vi "Start and Stop Sift Proxy.vi"() -> ()   [LabVIEW 2024]
uses:
  Sift API/Sift Client.lvclass
panel:
  out "Success":bool
  out "Count":i32
  out "Error":errorcluster
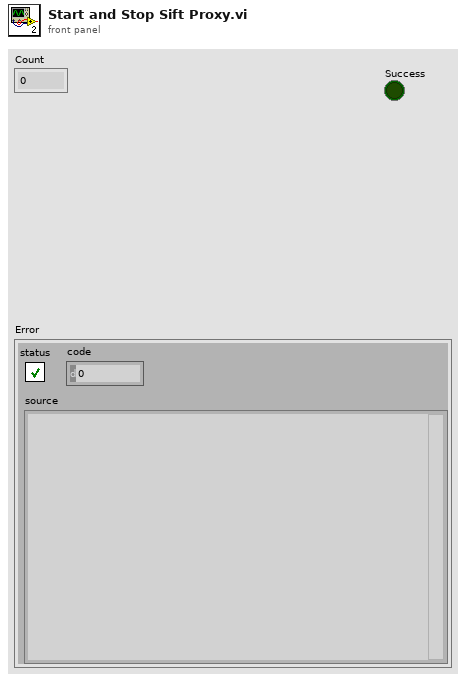
[diagram p1: front panel]
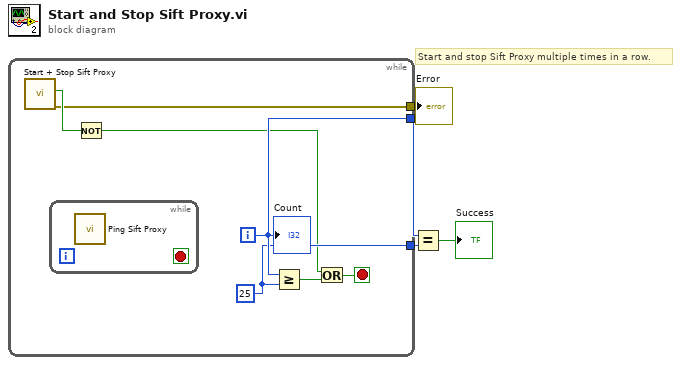
[diagram p0: block diagram]
diagram:
  # "Start and stop Sift Proxy multiple times in a row."
  n1 = while {
    tunnel: [w10] -> w4
    tunnel: [w9] -> w3
    tunnel: [w5] -> w1
    i -> [w10]
    stop <- w6 stop-if-true
    w9 = 25 ("x")
    n2 = call "Start + Stop Sift Proxy.vi"() -> ("Error"=w5:errorcluster, "Success"=w8:bool)  [unwired: 10 in]
    n3 = while {
      stop <- _ stop-if-true
      n4 = call-dynamic "Ping Sift Proxy.vi"() -> ()  [unwired: 13 in, 3 out]
    }
    n5 = Not(x=w8) -> (.not. x?=w7:bool)
    n6 = Greater Or Equal?(x=w10, y=w9) -> (x >= y?=w11:bool)
    n7 = Or(x=w7, y=w11) -> (x .or. y?=w6:bool)
    "Count" <- w10
  }
  "Error" <- w1
  n8 = Equal?(x=w4, y=w3) -> (x = y?=→"Success":bool)
